vi "CODCr质控流程 (子VI).vi"(9 "CODCr量程切换":enum32{"H", "L", "AUTO"}(ring)=enum."AUTO", 10 "CODCr":bool) -> (3 "布尔":bool)   [LabVIEW 2016, in "质控单元.lvlib"]
panel:
  out "CODCr中断报警":bool
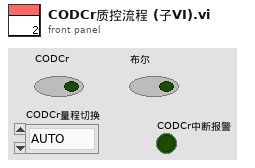
[diagram p1: front panel]
types:
  T1 = enum16{"待机", "启动水样测量", "水样测量中", "启动加标", "启动加标回收", "加标回收测量中", "结束"}
  T2 = cluster{"测量模式":enum16{"水样测量", "标样核查", "零点核查", "跨度核查", "空白测试", "加标回收", "平行样", "校零", "校标"}}
  T3 = enum16{"空闲", "水样测试", "标样核查", "零点核查", "跨度核查", "空白测试", "平行样测试", "加标回收", "空白校准", "标样校准", "初始化（清洗）"}
  T4 = cluster{"系统时间":timestamp, "工作状态":enum16{"空闲", "水样测试", "标样核查", "零点核查", "跨度核查", "空白测试", "平行样测试", "加标回收", "空白校准", "标样校准", "初始化（清洗）"}, "测量模式":enum16{"待机", "连续模式", "周期模式", "定点模式", "受控模式", "手动模式"}, "告警代码":enum16{"无告警", "缺试剂告警", "缺水样告警", "缺蒸馏水告警", "缺标液告警", "仪表漏液告警", "标定异常告警", "超量程告警", "加热异常", "低试剂预警", "超上限告警", "超下限告警", "仪表内部其他异常", "滴定异常告警", "电极异常告警", "量程切换告警", "参数设置告警", "PH电极电位异常", "电导率电极异常", "浊度光度异常", "溶解氧电极异常", "溶解氧光强异常", "温度异常告警", "PH异常告警", "溶解氧异常告警", "电导率异常告警", "浊度异常告警", "叶绿素异常告警", "藻密度异常告警", "蓝绿藻异常告警", "ORP异常告警", "氨氮异常告警", "清洁刷异常告警", "SD卡异常告警", "蓝牙异常告警", "Wifi异常告警", "流程异常告警"}, "故障代码":enum16{"无故障", "电机故障", "温度故障", "通讯故障", "滴定故障"}, "日志代码":u16, "软件版本":u16, "F0":sgl, "F1":sgl, "F2":sgl, "F3":sgl, "T":sgl, "H":sgl, "id":u16, "flowid":u16, "量程":u16, "总磷控温温度1":sgl, "营养盐控温温度2":sgl, "ADC":sgl}
  T5 = cluster{"因子编码":u32, "单位":u16, "标样参考值":sgl, "水样数据时间":timestamp, "水样实测值":sgl, "水样数据标识":string, "标样数据时间":timestamp, "标样实测值":sgl, "标样数据标识":string, "空白数据时间":timestamp, "空白实测值":sgl, "空白数据标识":string, "零点核查数据时间":timestamp, "零点核查实测值":sgl, "零点核查数据标识":string, "跨度核查数据时间":timestamp, "跨度核查实测值":sgl, "跨度核查数据标识":string, "加标回收数据时间":timestamp, "加标回收实测值":sgl, "加标回收数据标识":string, "平行样数据时间":timestamp, "平行样实测值":sgl, "平行样数据标识":string}
  T6 = cluster{"量程":dbl, "检出限":dbl, "加标前水样浓度":dbl, "加标后水样浓度":dbl, "加标水杯定容体积":dbl, "加标母液浓度":dbl, "加标体积":dbl, "加标回收率":dbl}
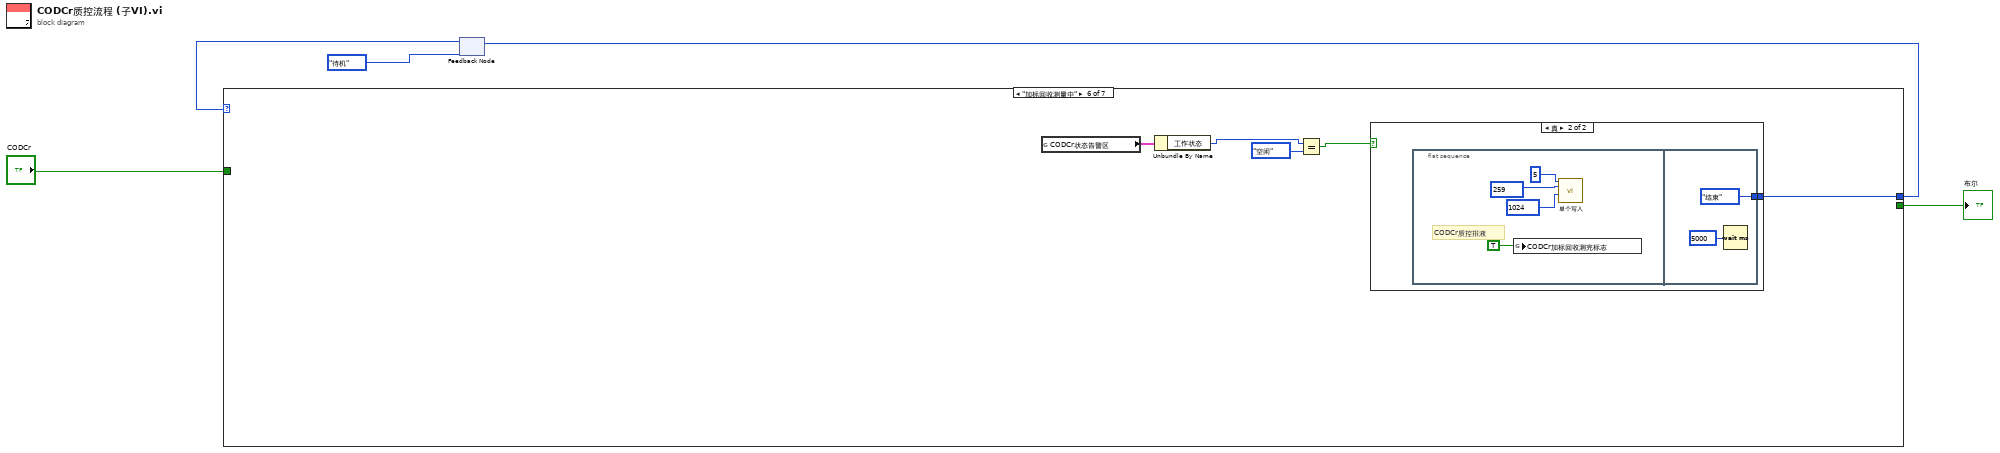
[diagram p0: block diagram]
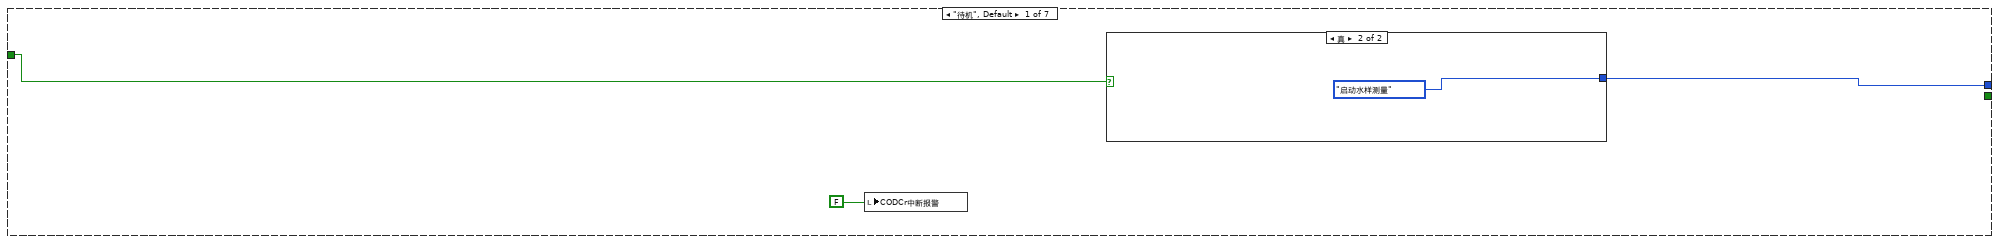
[diagram p2: hidden frame]
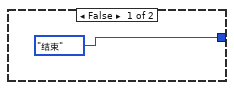
[diagram p3: hidden frame]
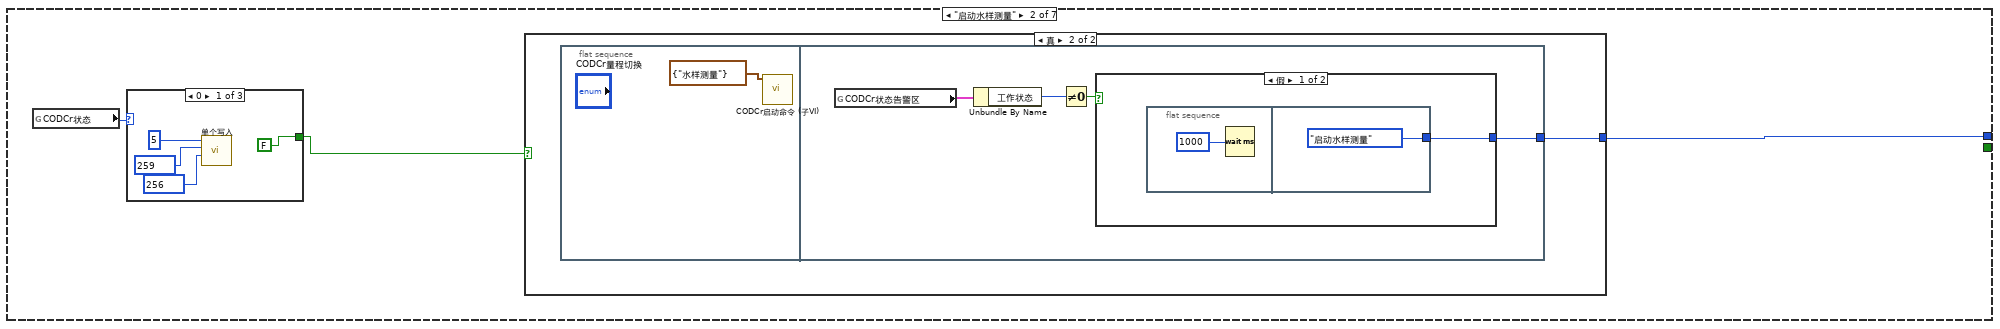
[diagram p4: hidden frame]
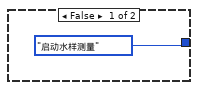
[diagram p5: hidden frame]
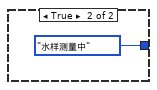
[diagram p6: hidden frame]
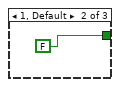
[diagram p7: hidden frame]
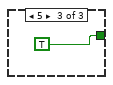
[diagram p8: hidden frame]
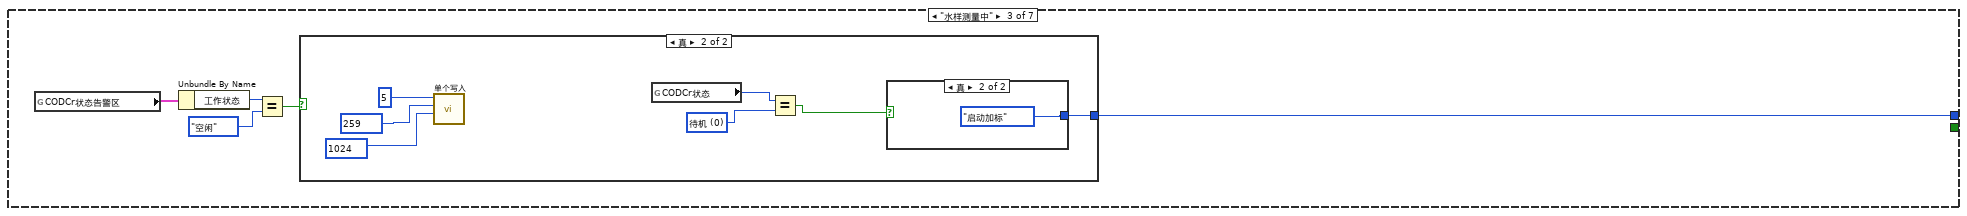
[diagram p9: hidden frame]
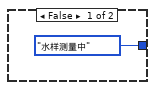
[diagram p10: hidden frame]
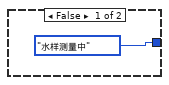
[diagram p11: hidden frame]
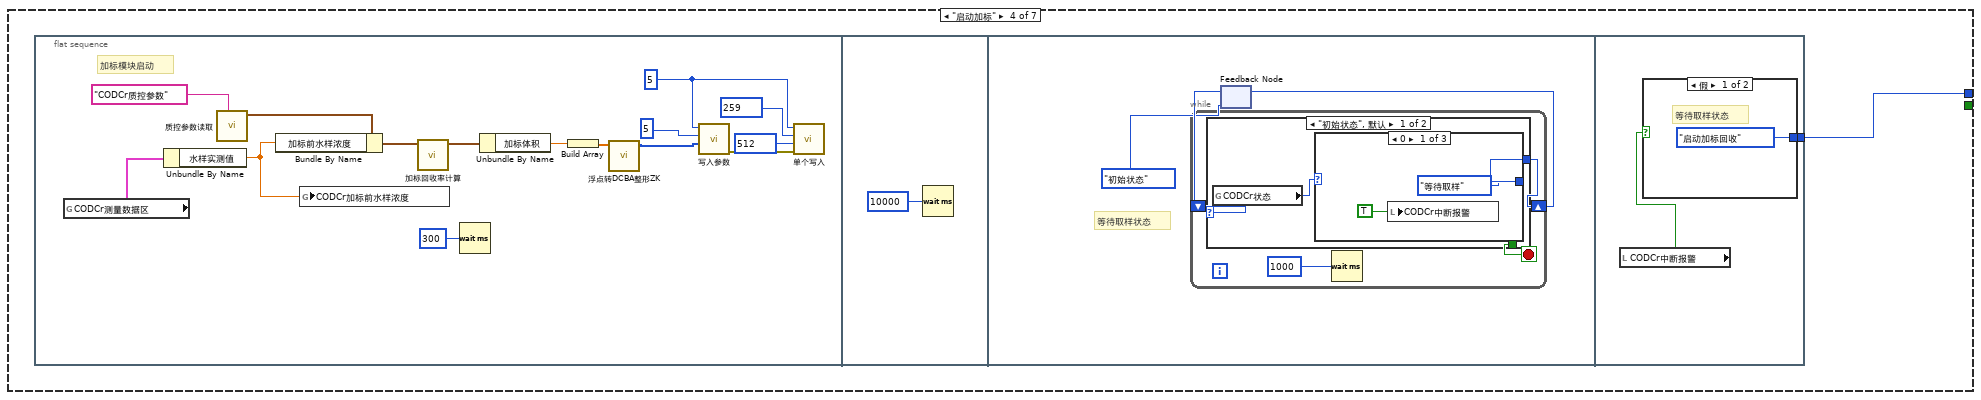
[diagram p12: hidden frame]
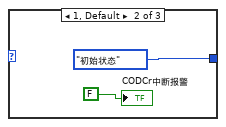
[diagram p13: hidden frame]
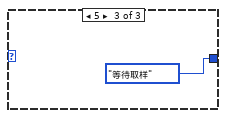
[diagram p14: hidden frame]
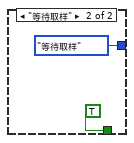
[diagram p15: hidden frame]
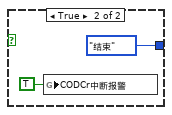
[diagram p16: hidden frame]
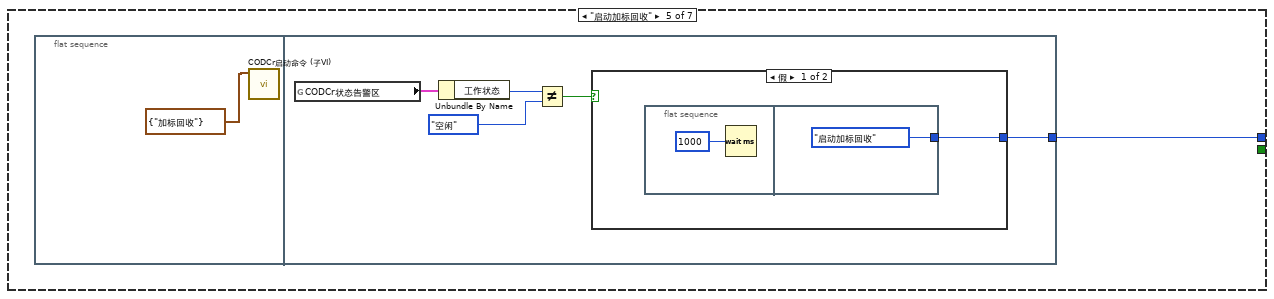
[diagram p17: hidden frame]
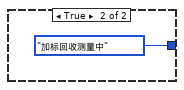
[diagram p18: hidden frame]
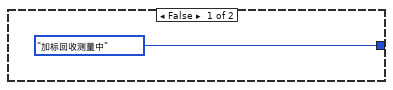
[diagram p19: hidden frame]
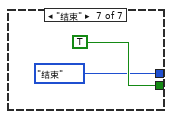
[diagram p20: hidden frame]
diagram:
  n1 = feedback #1(T1."待机") -> (w3:T1)
  n2 = case shown="\"加标回收测量中\"" w3 {
    tunnel: [w8 w13 w35 w46 w84 w99 T1."结束"] -> w4
    tunnel: [_ _ _ _ _ _ TRUE] -> w2
    tunnel: "CODCr" -> [w7 _ _ _ _ _ _]
    frame "待机", Default {
      n3 = local write "CODCr中断报警"(FALSE ("CODMn中断报警")) -> ()
      n4 = case shown="真" w7 {
        tunnel: [T1."结束" T1."启动水样测量"] -> w8
        frame False {
        }
        frame True {
        }
      }
    }
    frame "启动水样测量" {
      n5 = global read "加标回收状态全局变量.vi" "CODCr状态"() -> (w12:u16)
      n6 = case shown="0" w12 {
        tunnel: [FALSE ("s") FALSE ("s") TRUE ("s")] -> w11
        frame 0 {
          n7 = call "单个写入.vi"("value"=u16 256 ("starting address"), "address"=u16 259 ("starting address"), "Slave ID"=u8 5) -> ()  [unwired: 8 in, 1 out]
        }
        frame 1, Default {
        }
        frame 5 {
        }
      }
      n8 = case shown="真" w11 {
        tunnel: [T1."启动水样测量" w15] -> w13
        frame False {
        }
        frame True {
          n9 = flat-sequence {
            tunnel: [w20] -> w15
            frame #0 {
              n10 = call "CODCr启动命令 (子VI).vi"("启动测量模式"=T2 {"测量模式"=enum."水样测量"}) -> ()  [unwired: 10 in, 1 out]
            }
            frame #1 {
              n11 = global read "与CODCr交互全局.vi" "CODCr状态告警区"() -> (w18:T4)
              n12 = Unbundle By Name(w18) -> ("工作状态"=w19:T3)
              n13 = Not Equal To 0?(x=w19) -> (x != 0?=w17:bool)
              n14 = case shown="假" w17 {
                tunnel: [w21 T1."水样测量中"] -> w20
                frame False {
                  n15 = flat-sequence {
                    tunnel: [T1."启动水样测量"] -> w21
                    frame #0 {
                      n16 = Wait (ms)(milliseconds to wait=u32 1000 ("等待时间（毫秒）")) -> ()  [unwired: 1 out]
                    }
                    frame #1 {
                    }
                  }
                }
                frame True {
                }
              }
            }
          }
        }
      }
    }
    frame "水样测量中" {
      n17 = global read "与CODCr交互全局.vi" "CODCr状态告警区"() -> (w32:T4)
      n18 = Unbundle By Name(w32) -> ("工作状态"=w31:T3)
      n19 = Equal?(x=w31, y=T3."空闲") -> (x = y?=w33:bool)
      n20 = case shown="真" w33 {
        tunnel: [T1."水样测量中" w43] -> w35
        frame False {
        }
        frame True {
          w40 = u16 0 items=["待机", "润洗", "进样", "进样完成", "柱塞泵加标", "等待取液", "排液"] ("CODCr状态")
          n21 = call "单个写入.vi"("value"=u16 1024 ("starting address"), "address"=u16 259 ("starting address"), "Slave ID"=u8 5) -> ()  [unwired: 8 in, 1 out]
          n22 = global read "加标回收状态全局变量.vi" "CODCr状态"() -> (w41:u16)
          n23 = Equal?(x=w41, y=w40) -> (x = y?=w39:bool)
          n24 = case shown="真" w39 {
            tunnel: [T1."水样测量中" T1."启动加标"] -> w43
            frame False {
            }
            frame True {
            }
          }
        }
      }
    }
    frame "启动加标" {
      n25 = flat-sequence {
        tunnel: [w80] -> w46
        frame #0 {
          w54 = u16 5 ("value")
          # "加标模块启动"
          n26 = global read "与CODCr交互全局.vi" "CODCr测量数据区"() -> (w51:T5)
          n27 = Unbundle By Name(w51) -> ("水样实测值"=w52:sgl)
          n28 = call "质控参数读取.vi"("section"="CODCr质控参数") -> ("参数"=w59:T6)  [unwired: 9 in, 1 out]
          n29 = Bundle By Name(cluster=w59, "加标前水样浓度"=w52) -> (w60:T6)
          n30 = global write "水样浓度全局.vi" "CODCr加标前水样浓度"(w52) -> ()
          n31 = call "加标回收率计算.vi"("参数"=w60) -> ("参数 out"=w58:T6)  [unwired: 10 in]
          n32 = Wait (ms)(milliseconds to wait=u32 300 ("等待时间（毫秒）")) -> ()  [unwired: 1 out]
          n33 = Unbundle By Name(w58) -> ("加标体积"=w55:dbl)
          n34 = Build Array(w55) -> (w49:dbl[])
          n35 = call "浮点转DCBA整形ZK.vi"("浮点数"=w49) -> ("DCBA整形输出"=w50:u16[])  [unwired: 10 in]
          n36 = call "写入参数.vi"("values"=w50, "starting address"=u16 5, "Slave ID"=w54) -> ("error out"=w57:errorcluster)  [unwired: 8 in]
          n37 = call "单个写入.vi"("Error in"=w57, "value"=u16 512 ("starting address"), "address"=u16 259 ("starting address"), "Slave ID"=w54) -> ()  [unwired: 7 in, 1 out]
        }
        frame #1 {
          n38 = Wait (ms)(milliseconds to wait=u32 10000 ("等待时间（毫秒）")) -> ()  [unwired: 1 out]
        }
        frame #2 {
          # "等待取样状态"
          n39 = feedback #2(enum16{"初始状态", "等待取样"}."初始状态") -> (w64:enum16{"初始状态", "等待取样"})
          n40 = while {
            shift-right: [w68] -> w65
            shift-left: w64 -> [w69]
            stop <- w67 stop-if-true
            n41 = case shown="\"初始状态\", 默认" w69 {
              tunnel: [w71 enum16{"初始状态", "等待取样"}."等待取样"] -> w68
              tunnel: [_ TRUE] -> w67
              frame "初始状态", Default {
                n42 = global read "加标回收状态全局变量.vi" "CODCr状态"() -> (w70:u16)
                n43 = case shown="0" w70 {
                  tunnel: [enum16{"初始状态", "等待取样"}."等待取样" enum16{"初始状态", "等待取样"}."初始状态" enum16{"初始状态", "等待取样"}."等待取样"] -> w71
                  frame 0 {
                    n44 = local write "CODCr中断报警"(TRUE ("氨氮中断报警")) -> ()
                  }
                  frame 1, Default {
                    "CODCr中断报警" <- FALSE ("总氮中断报警")
                  }
                  frame 5 {
                  }
                }
              }
              frame "等待取样" {
              }
            }
            n45 = Wait (ms)(milliseconds to wait=u32 1000 ("等待时间（毫秒）")) -> ()  [unwired: 1 out]
          }
          n46 = feedback-in #2(w65) -> ()
        }
        frame #3 {
          n47 = local read "CODCr中断报警"() -> (w79:bool)
          n48 = case shown="假" w79 {
            tunnel: [T1."启动加标回收" T1."结束"] -> w80
            frame False {
              # "等待取样状态"
            }
            frame True {
              n49 = global write "质控中断报警全局.vi" "CODCr中断报警"(TRUE ("CODCr中断报警")) -> ()
            }
          }
        }
      }
    }
    frame "启动加标回收" {
      n50 = flat-sequence {
        tunnel: [w90] -> w84
        frame #0 {
          n51 = call "CODCr启动命令 (子VI).vi"("启动测量模式"=T2 {"测量模式"=enum."加标回收"}) -> ()  [unwired: 10 in, 1 out]
        }
        frame #1 {
          n52 = global read "与CODCr交互全局.vi" "CODCr状态告警区"() -> (w89:T4)
          n53 = Unbundle By Name(w89) -> ("工作状态"=w88:T3)
          n54 = Not Equal?(x=w88, y=T3."空闲") -> (x != y?=w86:bool)
          n55 = case shown="假" w86 {
            tunnel: [w91 T1."加标回收测量中"] -> w90
            frame False {
              n56 = flat-sequence {
                tunnel: [T1."启动加标回收"] -> w91
                frame #0 {
                  n57 = Wait (ms)(milliseconds to wait=u32 1000 ("等待时间（毫秒）")) -> ()  [unwired: 1 out]
                }
                frame #1 {
                }
              }
            }
            frame True {
            }
          }
        }
      }
    }
    frame "加标回收测量中" {
      n58 = global read "与CODCr交互全局.vi" "CODCr状态告警区"() -> (w96:T4)
      n59 = Unbundle By Name(w96) -> ("工作状态"=w95:T3)
      n60 = Equal?(x=w95, y=T3."空闲") -> (x = y?=w97:bool)
      n61 = case shown="真" w97 {
        tunnel: [T1."加标回收测量中" w101] -> w99
        frame False {
        }
        frame True {
          n62 = flat-sequence {
            tunnel: [T1."结束"] -> w101
            frame #0 {
              # "CODCr质控排液"
              n63 = global write "质控测完标志全局 1.vi" "CODCr加标回收测完标志"(TRUE ("COD加标回收测完标志")) -> ()
              n64 = call "单个写入.vi"("value"=u16 1024 ("starting address"), "address"=u16 259 ("starting address"), "Slave ID"=u8 5) -> ()  [unwired: 8 in, 1 out]
            }
            frame #1 {
              n65 = Wait (ms)(milliseconds to wait=u32 5000 ("等待时间（毫秒）")) -> ()  [unwired: 1 out]
            }
          }
        }
      }
    }
    frame "结束" {
    }
  }
  "布尔" <- w2
  n66 = feedback-in #1(w4) -> ()
